vi "Decode MUS.vi"(8 "error in":errorcluster, 11 "Music_Lump in":u8[](array[numeric])) -> (0 "error out":errorcluster, 2 "midi_Msg":u32[](array[numeric]) format="%x", 3 "delay":u32[](array[numeric]))   [LabVIEW 2014]
panel:
  out "MUS event value":u8[](array[numeric]) format="%.0b"
  in  "Vol_temp":u8=127
  out "CH_totl":u16
  out "event size":i32
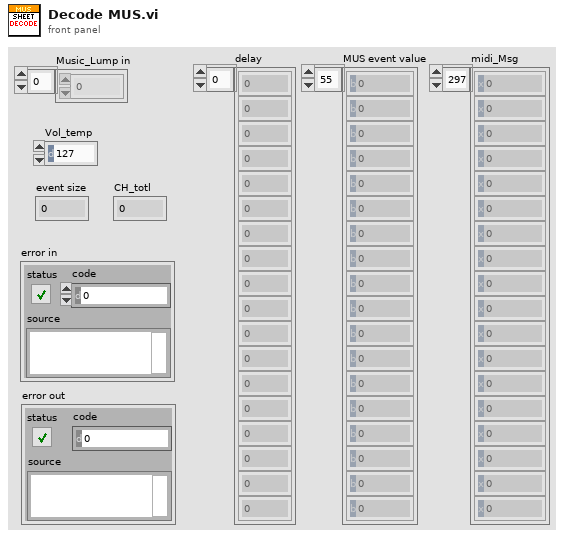
[diagram p1: front panel]
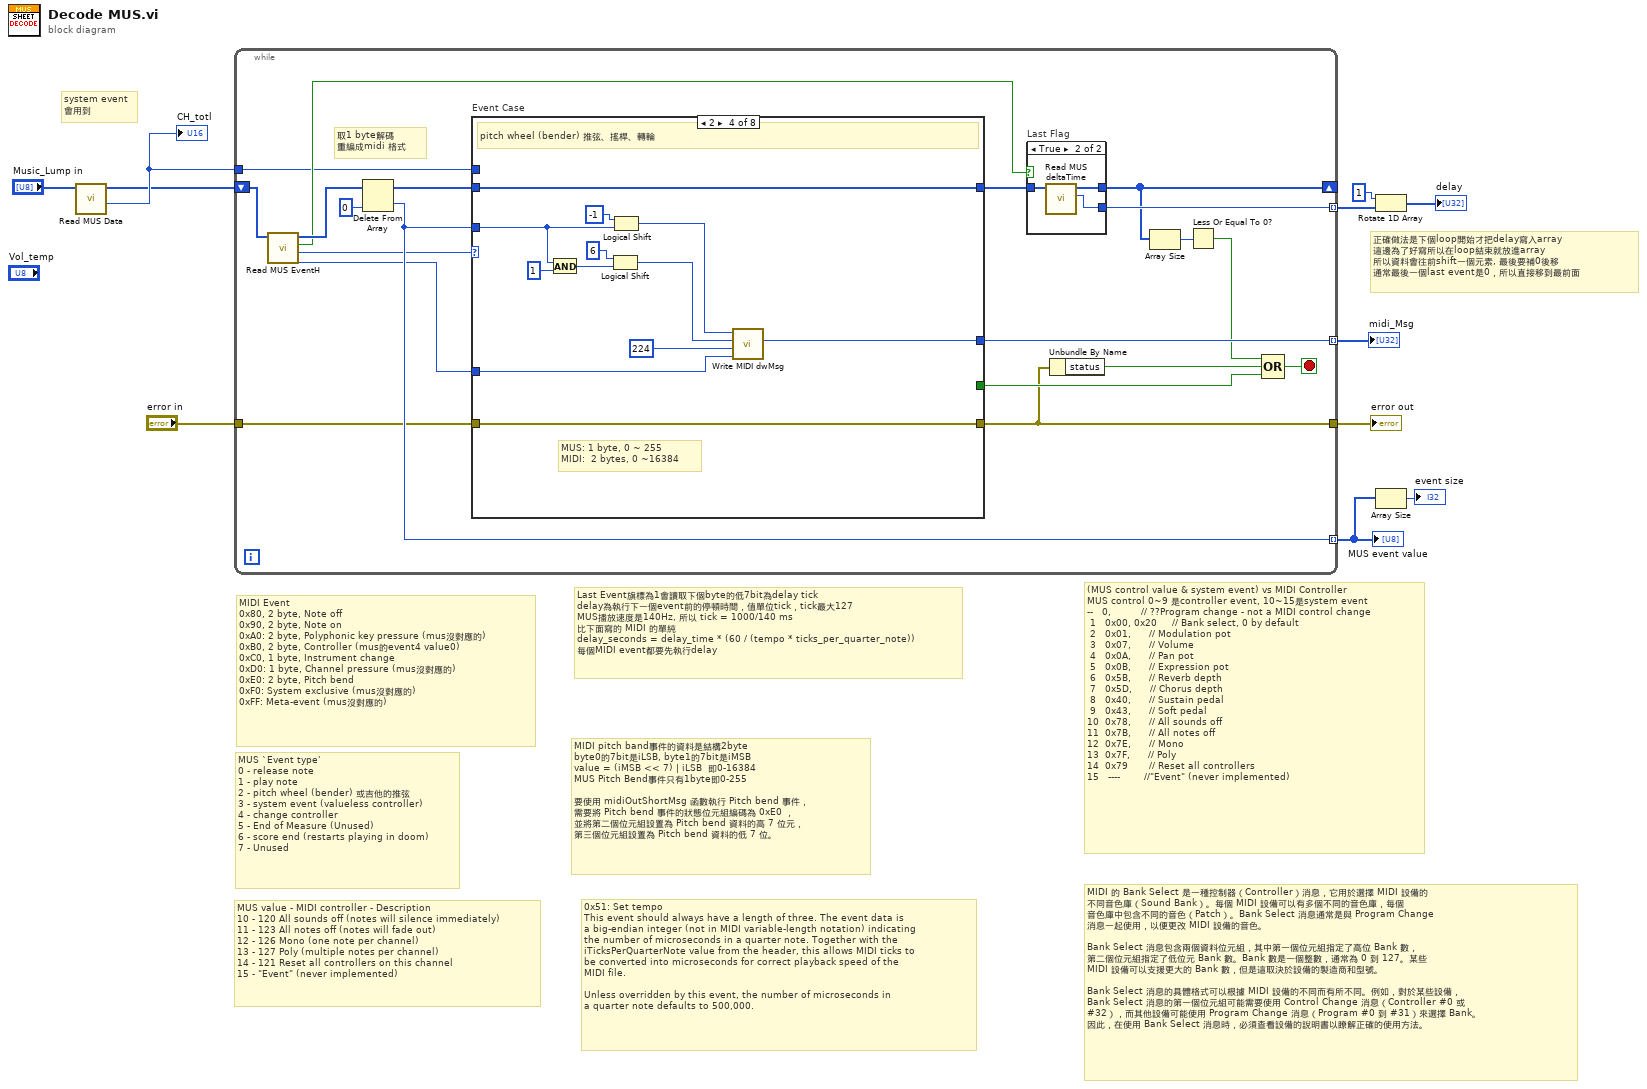
[diagram p0: block diagram]
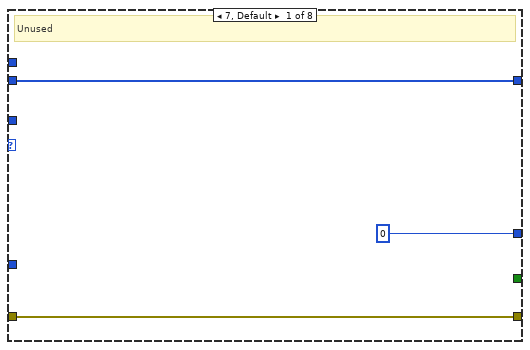
[diagram p2: hidden frame]
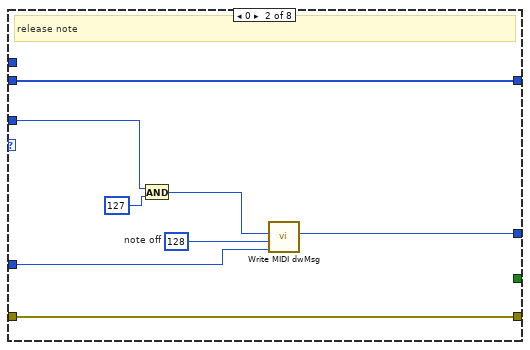
[diagram p3: hidden frame]
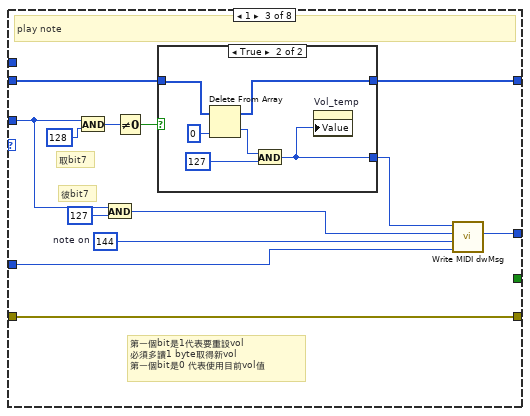
[diagram p4: hidden frame]
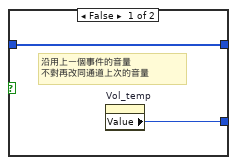
[diagram p5: hidden frame]
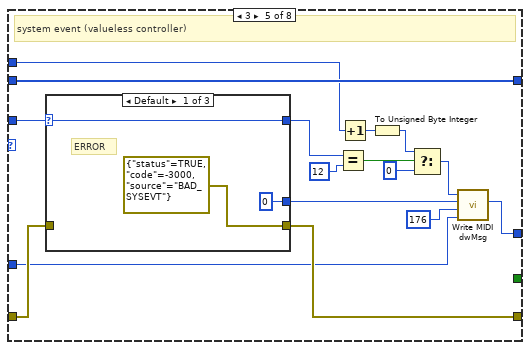
[diagram p6: hidden frame]
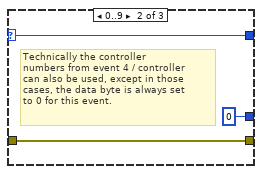
[diagram p7: hidden frame]
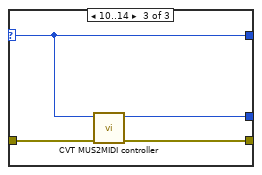
[diagram p8: hidden frame]
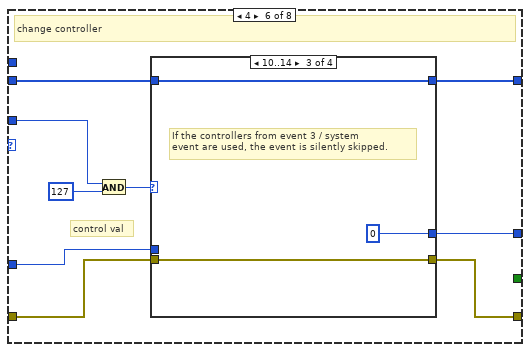
[diagram p9: hidden frame]
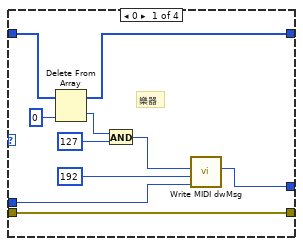
[diagram p10: hidden frame]
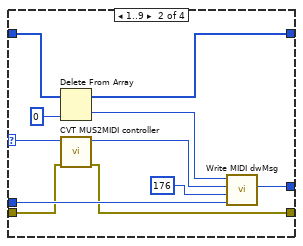
[diagram p11: hidden frame]
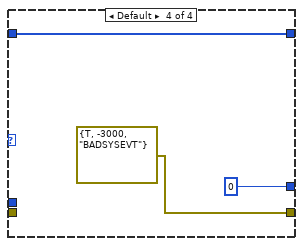
[diagram p12: hidden frame]
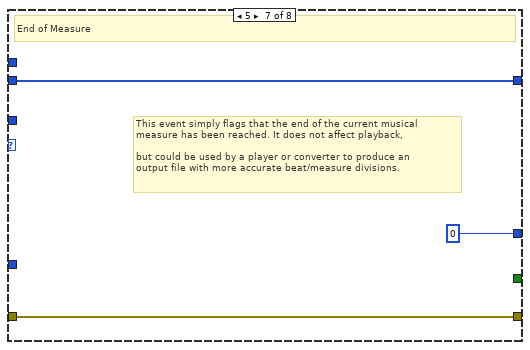
[diagram p13: hidden frame]
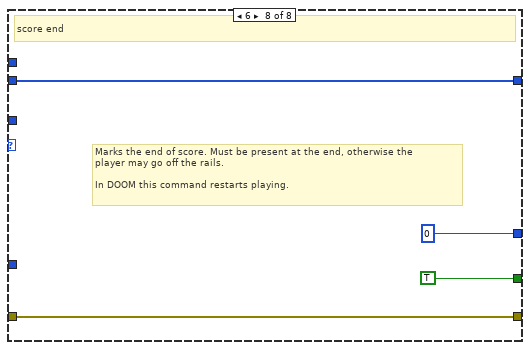
[diagram p14: hidden frame]
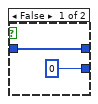
[diagram p15: hidden frame]
diagram:
  # "MUS value - MIDI controller - Description\n10 - 120\tAll sounds off (notes will silence immediately)\n11\t- 123\tAll notes off (notes will fade out)\n12\t- 126\tMono (one note per channel)\n13\t- 127\tPoly (multiple notes per channel)\n14\t- 121\tReset all controllers on this channel\n15\t-\t\"Event\" (never implemented)"
  # "0x51: Set tempo\nThis event should always have a length of three. The event data is \na big-endian integer (not in MIDI variable-length notation) indicating \nthe number of microseconds in a quarter note. Together with the \niTicksPerQuarterNote value from the header, this allows MIDI ticks to \nbe converted into microseconds for correct playback speed of the \nMIDI file.\n\nUnless overridden by this event, the number of microseconds in \na quarter note defaults to 500,000."
  # "system event\n會用到"
  # "正確做法是下個loop開始才把delay寫入array\n這邊為了好寫所以在loop結束就放進array\n所以資料會往前shift一個元素, 最後要補0後移\n通常最後一個last event是0，所以直接移到最前面"
  # "MIDI pitch band事件的資料是結構2byte\nbyte0的7bit是iLSB, byte1的7bit是iMSB\nvalue = (iMSB << 7) | iLSB  即0-16384\nMUS Pitch Bend事件只有1byte即0-255\n\n要使用 midiOutShortMsg 函數執行 Pitch bend 事件，\n需要將 Pitch bend 事件的狀態位元組編碼為 0xE0 ，\n並將第二個位元組設置為 Pitch bend 資料的高 7 位元，\n第三個位元組設置為 Pitch bend 資料的低 7 位。"
  # "Last Event旗標為1會讀取下個byte的低7bit為delay tick\ndelay為執行下一個event前的停頓時間，值單位tick，tick最大127\nMUS播放速度是140Hz, 所以 tick = 1000/140 ms\n比下面寫的 MIDI 的單純\ndelay_seconds = delay_time * (60 / (tempo * ticks_per_quarter_note))\n每個MIDI event都要先執行delay"
  # "MUS `Event type'\n0 - release note\n1 - play note\n2 - pitch wheel (bender) 或吉他的推弦\n3 - system event (valueless controller)\n4 - change controller\n5 - End of Measure (Unused)\n6 - score end (restarts playing in doom)\n7 - Unused"
  # "MIDI 的 Bank Select 是一種控制器（Controller）消息，它用於選擇 MIDI 設備的\n不同音色庫（Sound Bank）。每個 MIDI 設備可以有多個不同的音色庫，每個\n音色庫中包含不同的音色（Patch）。Bank Select 消息通常是與 Program Change \n消息一起使用，以便更改 MIDI 設備的音色。\n\nBank Select 消息包含兩個資料位元組，其中第一個位元組指定了高位 Bank 數，\n第二個位元組指定了低位元 Bank 數。Bank 數是一個整數，通常為 0 到 127。某些 \nMIDI 設備可以支援更大的 Bank 數，但是這取決於設備的製造商和型號。\n\nBank Select 消息的具體格式可以根據 MIDI 設備的不同而有所不同。例如，對於某些設備，\nBank Select 消息的第一個位元組可能需要使用 Control Change 消息（Controller #0 或 \n#32），而其他設備可能使用 Program Change 消息（Program #0 到 #31）來選擇 Bank。\n因此，在使用 Bank Select 消息時，必須查看設備的說明書以瞭解正確的使用方法。"
  # "MIDI Event\n0x80, 2 byte, Note off \n0x90, 2 byte, Note on\n0xA0: 2 byte, Polyphonic key pressure (mus沒對應的) \n0xB0, 2 byte, Controller (mus的event4 value0) \n0xC0, 1 byte, Instrument change\n0xD0: 1 byte, Channel pressure (mus沒對應的) \n0xE0: 2 byte, Pitch bend \n0xF0: System exclusive (mus沒對應的) \n0xFF: Meta-event (mus沒對應的)"
  # "(MUS control value & system event) vs MIDI Controller \nMUS control 0~9 是controller event, 10~15是system event\n--   0,          // ??Program change - not a MIDI control change\n 1   0x00, 0x20     // Bank select, 0 by default\n 2   0x01,      // Modulation pot\n 3   0x07,      // Volume\n 4   0x0A,      // Pan pot\n 5   0x0B,      // Expression pot\n 6   0x5B,      // Reverb depth\n 7   0x5D,      // Chorus depth\n 8   0x40,      // Sustain pedal\n 9   0x43,      // Soft pedal\n10  0x78,      // All sounds off\n11  0x7B,      // All notes off\n12  0x7E,      // Mono\n13  0x7F,      // Poly\n14  0x79       // Reset all controllers\n15   ----        //\"Event\" (never implemented)"
  n1 = call "Read MUS Data.vi"("Sound LUMP IN"="Music_Lump in") -> ("CHAN_total"=w10:u16, "MUS_Data_out"=w4:u8[])  [unwired: 7 in, 2 out]
  "CH_totl" <- w10
  n2 = while {
    shift-right: [w24] -> _
    shift-left: w4 -> [w31]
    tunnel: [w26] -> w5 mode=indexing
    tunnel: [w25] -> w6 mode=indexing
    tunnel: [w21] -> w1 mode=indexing
    tunnel: w10 -> [w16]
    tunnel: "error in" -> [w15]
    tunnel: [w13] -> w2
    stop <- w17 stop-if-true
    # "取1 byte解碼\n重編成midi 格式"
    n3 = call "Read MUS EventH.vi"("MUS_Data_in"=w31) -> ("CAHN"=w20:u8, "Even_No"=w14:u8, "Last flag?"=w22:bool, "Data_Remaining"=w30:u8[])  [unwired: 7 in]
    n4 = Delete From Array(array=w30, index=0) -> (deleted portion=w21:u8, array with subset deleted=w29:u8[])  [unwired: 1 in]
    n5 = case "Event Case" shown="2" w14 {
      tunnel: [_ _ _ _ _ _ _ TRUE] -> w18
      tunnel: [w34 w41 w50 w74 w91 w105 w140 w143] -> w27
      tunnel: w20 -> [_ w36 w45 w64 w76 w102 _ _]
      tunnel: [u32 0 ("event_dwMsg") w38 w47 w66 w80 w108 u32 0 ("event_dwMsg") u32 0 ("event_dwMsg")] -> w26
      tunnel: w29 -> [w34 w41 w51 w74 w91 w106 w140 w143]
      tunnel: w21 -> [_ w40 w53 w70 w90 w109 _ _]
      tunnel: [w32 w37 w46 w65 w79 w104 w138 w141] -> w13
      tunnel: w16 -> [_ _ _ _ w78 _ _ _]
      tunnel: w15 -> [w32 w37 w46 w65 w77 w103 w138 w141]
      frame 7, Default {
        # "Unused"
      }
      frame 0 {
        w39 = u8 128  # note off
        # "release note"
        n6 = And(x=w40, y=u8 127) -> (x .and. y?=w35:u8)
        n7 = call "Write MIDI dwMsg.vi"("channel"=w36, "MIDI_event"=w39, "lo_byte"=w35) -> ("event_dwMsg"=w38:u32)  [unwired: 8 in]
      }
      frame 1 {
        w48 = u8 144  # note on
        # "第一個bit是1代表要重設vol\n必須多讀1 byte取得新vol\n第一個bit是0 代表使用目前vol值"
        # "彼bit7"
        # "取bit7"
        # "play note"
        n8 = And(x=w53, y=u8 128) -> (x .and. y?=w52:u8)
        n9 = And(x=w53, y=u8 127) -> (x .and. y?=w43:u8)
        n10 = Not Equal To 0?(x=w52) -> (x != 0?=w49:bool)
        n11 = case shown="True" w49 {
          tunnel: w51 -> [w57 w62]
          tunnel: [w57 w61] -> w50
          tunnel: [w56 w58] -> w44
          frame False {
            # "沿用上一個事件的音量\n不對再改同通道上次的音量"
            n12 = property on="Vol_temp" class="DigNum (strict)"() -> ("Value"=w56:u8)  [unwired: 2 in, 2 out]
          }
          frame True {
            n13 = Delete From Array(array=w62, index=0) -> (deleted portion=w59:u8, array with subset deleted=w61:u8[])  [unwired: 1 in]
            n14 = And(x=w59, y=u8 127) -> (x .and. y?=w58:u8)
            n15 = property on="Vol_temp" class="DigNum (strict)"("Value"=w58) -> ()  [unwired: 2 in, 2 out]
          }
        }
        n16 = call "Write MIDI dwMsg.vi"("channel"=w45, "MIDI_event"=w48, "lo_byte"=w43, "hi_byte"=w44) -> ("event_dwMsg"=w47:u32)  [unwired: 7 in]
      }
      frame 2 {
        # "MUS: 1 byte, 0 ~ 255\nMIDI:  2 bytes, 0 ~16384"
        # "pitch wheel (bender) 推弦、搖桿、轉輪"
        n17 = And(x=w70, y=u8 1) -> (x .and. y?=w73:u8)
        n18 = Logical Shift(y=i16 6, x=w73) -> (x << y=w68:u8)
        n19 = Logical Shift(y=i16 -1, x=w70) -> (x << y=w67:u8)
        n20 = call "Write MIDI dwMsg.vi"("channel"=w64, "MIDI_event"=u8 224 ("data"), "lo_byte"=w68, "hi_byte"=w67) -> ("event_dwMsg"=w66:u32)  [unwired: 7 in]
      }
      frame 3 {
        # "system event (valueless controller)"
        n21 = case shown="Default" w90 {
          selector: w90 -> [w93 w96 w100]
          tunnel: [u8 0 u8 0 w101] -> w82
          tunnel: [w93 w96 w100] -> w88
          tunnel: [errorcluster {"status"=TRUE, "code"=-3000, "source"="BAD_SYSEVT"} ("error constant") w95 w98] -> w79
          tunnel: w77 -> [_ w95 w99]
          frame Default {
            # "ERROR"
          }
          frame 0..9 {
            # "Technically the controller \nnumbers from event 4 / controller \ncan also be used, except in those \ncases, the data byte is always set \nto 0 for this event."
          }
          frame 10..14 {
            n22 = call "CVT MUS2MIDI controller.vi"("error in"=w99, "MSU set"=w100) -> ("error out"=w98:errorcluster, "midi_ctrl"=w101:u8)  [unwired: 8 in]
          }
        }
        n23 = Equal?(x=w88, y=u8 12) -> (x = y?=w87:bool)
        n24 = Increment(x=w78) -> (x+1=w86:u16)
        n25 = To Unsigned Byte Integer(number=w86) -> (unsigned 8bit integer=w85:u8)
        n26 = Select(t=w85, s=w87, f=u8 0) -> (s? t:f=w83:u8)
        n27 = call "Write MIDI dwMsg.vi"("channel"=w76, "MIDI_event"=u8 176 ("data"), "lo_byte"=w82, "hi_byte"=w83) -> ("event_dwMsg"=w80:u32)  [unwired: 7 in]
      }
      frame 4 {
        # "control val"
        # "change controller"
        n28 = And(x=w109, y=u8 127) -> (x .and. y?=w107:u8)
        n29 = case shown="10..14" w107 {
          selector: w107 -> [_ w128 _ _]
          tunnel: w102 -> [w113 w123 _ _]
          tunnel: [w112 w127 u32 0 u32 0] -> w108
          tunnel: w106 -> [w118 w131 w133 w136]
          tunnel: [w116 w130 w133 w136] -> w105
          tunnel: [w111 w121 w132 errorcluster {"status"=TRUE, "code"=-3000, "source"="BADSYSEVT"} ("error constant")] -> w104
          tunnel: w103 -> [w111 w122 w132 _]
          frame 0 {
            # "樂器"
            n30 = Delete From Array(array=w118, index=0) -> (deleted portion=w117:u8, array with subset deleted=w116:u8[])  [unwired: 1 in]
            n31 = And(x=w117, y=u8 127) -> (x .and. y?=w115:u8)
            n32 = call "Write MIDI dwMsg.vi"("channel"=w113, "MIDI_event"=u8 192 ("data"), "lo_byte"=w115) -> ("event_dwMsg"=w112:u32)  [unwired: 8 in]
          }
          frame 1..9 {
            n33 = Delete From Array(array=w131, index=0) -> (deleted portion=w126:u8, array with subset deleted=w130:u8[])  [unwired: 1 in]
            n34 = call "CVT MUS2MIDI controller.vi"("error in"=w122, "MSU set"=w128) -> ("error out"=w121:errorcluster, "midi_ctrl"=w125:u8)  [unwired: 8 in]
            n35 = call "Write MIDI dwMsg.vi"("channel"=w123, "MIDI_event"=u8 176 ("data"), "lo_byte"=w125, "hi_byte"=w126) -> ("event_dwMsg"=w127:u32)  [unwired: 7 in]
          }
          frame 10..14 {
            # "If the controllers from event 3 / system \nevent are used, the event is silently skipped."
          }
          frame Default {
          }
        }
      }
      frame 5 {
        # "This event simply flags that the end of the current musical \nmeasure has been reached. It does not affect playback, \n\nbut could be used by a player or converter to produce an \noutput file with more accurate beat/measure divisions."
        # "End of Measure"
      }
      frame 6 {
        # "Marks the end of score. Must be present at the end, otherwise the\nplayer may go off the rails. \n\nIn DOOM this command restarts playing."
        # "score end"
      }
    }
    n36 = case "Last Flag" shown="True" w22 {
      tunnel: w27 -> [w146 w149]
      tunnel: [w146 w148] -> w24
      tunnel: [u32 0 ("delay") w147] -> w25
      frame False {
      }
      frame True {
        n37 = call "Read MUS deltaTime.vi"("MUS_Data_in"=w149) -> ("delay_tick"=w147:u32, "Data_Remaining"=w148:u8[])  [unwired: 9 in]
      }
    }
    n38 = Unbundle By Name(w13) -> ("status"=w12:bool)
    n39 = Array Size(array=w24) -> (size(s)=w23:i32)
    n40 = Less Or Equal To 0?(x=w23) -> (x <= 0?=w19:bool)
    n41 = Compound Arithmetic op=OR(w19, w12, w18) -> (w17:bool)
  }
  "midi_Msg" <- w5
  "MUS event value" <- w1
  "error out" <- w2
  n42 = Rotate 1D Array(1:w6, 2:1 ("n")) -> (0:→"delay":u32[])
  n43 = Array Size(array=w1) -> (size(s)=→"event size":i32)
